vi "Remove Duplicates Colors.vi"(0 "Input Array":u32[](array[numeric])) -> (1 "Output Array":u32[](array[numeric]), 2 "indices of removed elements":i32[](array[numeric]))   [LabVIEW 2020, in "PieChart.lvclass"]
doc: "<b> </b> <b> </b>\n©2013, Q Software Innovations, LLC.\n\nWritten in National Instruments LabVIEW™ 2013.\n\nAuthored by Quentin Alldredge\nQ@qsoftwareinnovations.com\nwww.qsoftwareinnovations.com\n\nAll rights reserved."
uses:
  PieChart.lvclass
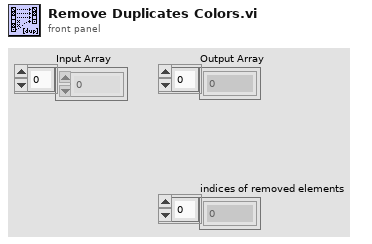
[diagram p1: front panel]
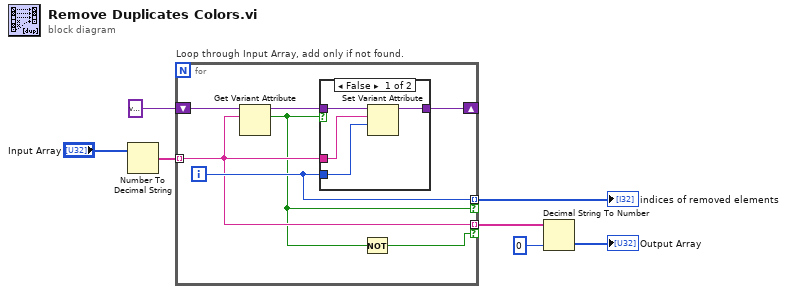
[diagram p0: block diagram]
diagram:
  n1 = Number To Decimal String(number="Input Array") -> (decimal integer string=w4:string[])  [unwired: 1 in]
  n2 = for "Loop through Input Array, add only if not found." {
    shift-right: [w14] -> _
    shift-left: variant -> [w13]
    tunnel: w4 -> [w10] mode=indexing
    tunnel: [w11] -> w1 mode=indexing if=w9
    tunnel: [w10] -> w3 mode=indexing if=w8
    i -> [w11]
    n3 = Get Variant Attribute(Variant=w13, name=w10) -> (duplicate Variant=w12:variant, found=w9:bool)  [unwired: 2 in, 2 out]
    n4 = case shown="False" w9 {
      tunnel: [w18 w19] -> w14
      tunnel: w10 -> [w17 _]
      tunnel: w12 -> [w16 w19]
      tunnel: w11 -> [w15 _]
      frame False {
        n5 = Set Variant Attribute(Variant=w16, name=w17, value=w15) -> (Variant out=w18:variant)  [unwired: 1 in, 2 out]
      }
      frame True {
      }
    }
    n6 = Not(x=w9) -> (.not. x?=w8:bool)
  }
  "indices of removed elements" <- w1
  n7 = Decimal String To Number(string=w3, default (0L)=u32 0 ("default (0 I32)")) -> (number=→"Output Array":u32[])  [unwired: 1 in, 1 out]
